vi "uActor_Stall_Caller.vi"(7 "checking rate (250 ms)":u32=250, 8 "error in (no error)":errorcluster, 11 "uActor Transport":refnum<class "uTransport_uActor.lvclass">) -> (0 "error out":errorcluster)   [LabVIEW 2023, in "uFramework.lvlib" / "uActor.lvclass"]
doc: "Stall until the actor stops. This is used to keep the caller VI in a 'running' state as long as the actor is still alive."
uses:
  uActor.lvclass
  uTransport_uActor/uTransport_uActor.lvclass
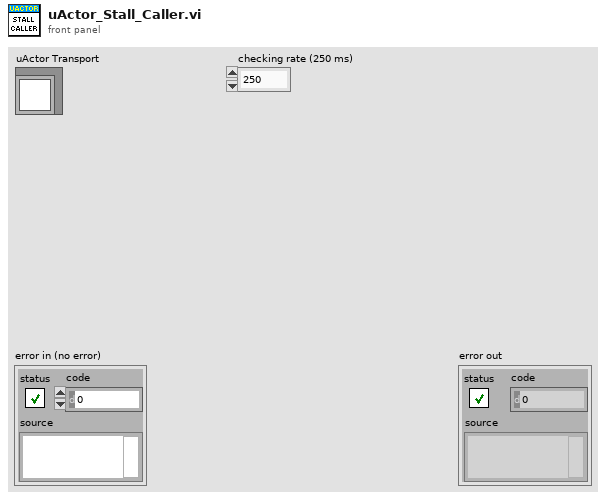
[diagram p1: front panel]
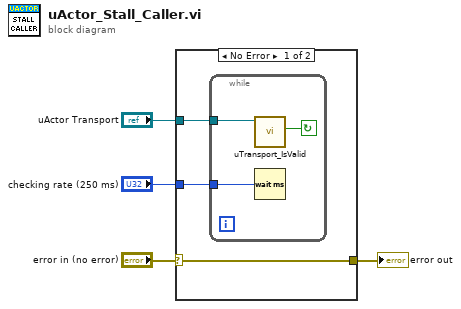
[diagram p0: block diagram]
diagram:
  n1 = case shown="No Error" "error in (no error)" {
    selector: "error in (no error)" -> [w7 w11]
    tunnel: [w7 w11] -> w3
    tunnel: "uActor Transport" -> [w6 _]
    tunnel: "checking rate (250 ms)" -> [w5 _]
    frame No Error {
      n2 = while {
        tunnel: w6 -> [w10]
        tunnel: w5 -> [w8]
        stop <- w9 continue-if-true
        n3 = call-dynamic "uTransport_IsValid.vi"("uTransport_uActor in"=w10) -> ("IsValid?"=w9:bool)  [unwired: 8 in, 2 out]
        n4 = Wait (ms)(milliseconds to wait=w8) -> ()  [unwired: 1 out]
      }
    }
    frame Error {
    }
  }
  "error out" <- w3
